vi "Convert Seconds to Milliseconds.vi"(11 "Time (sec)":dbl) -> (3 "Time (ms)":i32)   [LabVIEW 2020, in "ChromTech Next Gen Pump.lvlib" / "Acquisition.lvlib"]
uses:
  Acquisition.lvlib
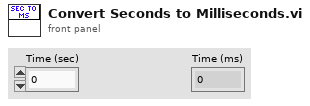
[diagram p1: front panel]
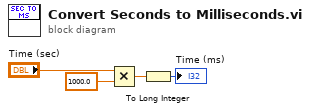
[diagram p0: block diagram]
diagram:
  n1 = Multiply(x="Time (sec)", y=1000.0) -> (x*y=w3:dbl)
  n2 = To Long Integer(number=w3) -> (32bit integer=→"Time (ms)":i32)
